vi "Fetch Digital Waveform.vi"(8 "error in (no error)":errorcluster, 9 "Timeout (10000 ms)":u32=10000, 10 "Source (0: POD 1)":u16(ring) items=["POD 1", "POD 2"], 11 "VISA resource name":refnum<visa-resource-name>) -> (0 "error out":errorcluster, 2 "Digital Waveform Graph":digitalwaveform(graph), 3 "VISA resource name out":refnum<visa-resource-name>)   [LabVIEW 2018, in "Agilent 6000 Series.lvlib"]
doc: "Returns the waveform the oscilloscope acquired for the specified channel. The waveform is from an acquisition that you initiate prior to calling this VI.\n\nYou use the Initiate VI to start an acquisition on the channels that you enable with the <B>Configure Digital Channel</B> VI. The oscilloscope acquires waveforms for the enabled channels concurrently. You must call this VI separately for each enabled channel to obtain the waveforms.\n\nYou can call the <B>Read Digital Waveform</B> VI instead of using low level VIs.\n\n<B>NOTE:</B>\n\n1. This VI is only supported by MSO models; running this VI with a DSO model might throw an error.\n\n2. This VI does not check the instrument status. Typically, you call this VI only in a sequence of calls to other low-level instrument driver VIs. The sequence performs one operation. You use the low-level VIs to optimize one or more aspects of interaction with the instrument."
uses:
  Agilent 6000 Series.lvlib
  <vilib>/Waveform/DWDTOps.llb/DWDT Boolean Array to Digital.vi
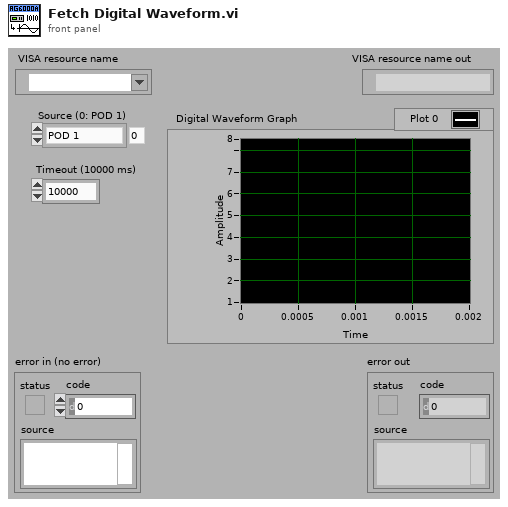
[diagram p1: front panel]
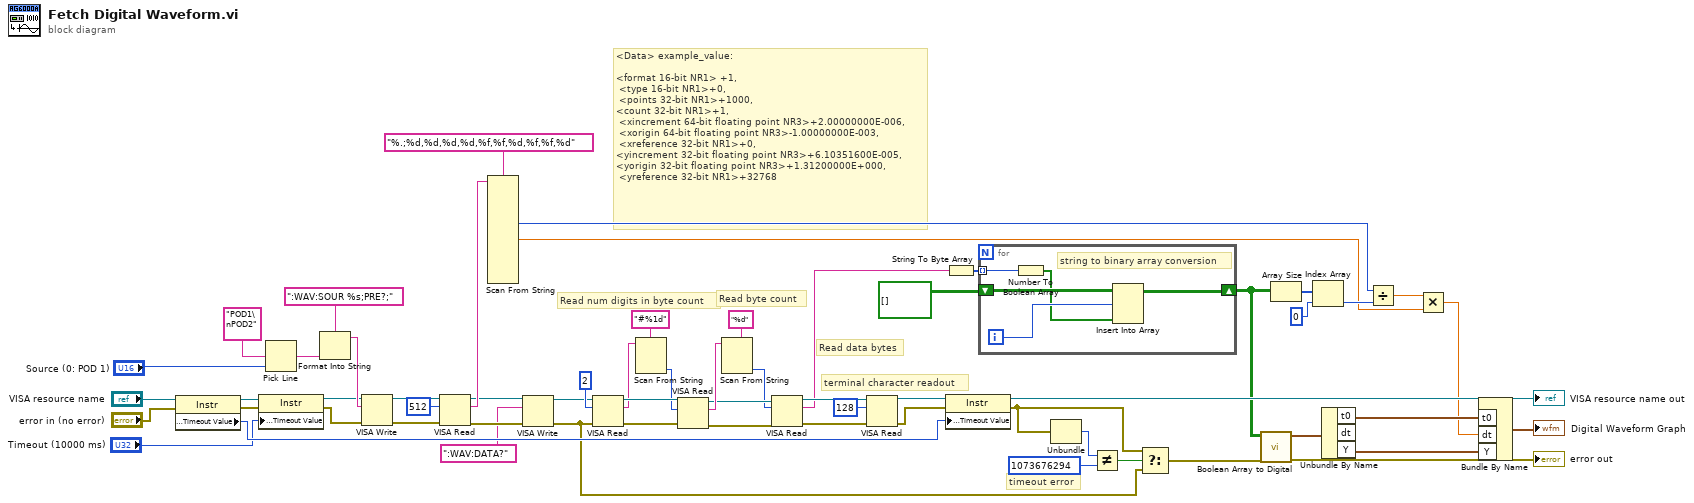
[diagram p0: block diagram]
diagram:
  # "timeout error"
  # "<Data> example_value:\n\n<format 16-bit NR1> +1,\n <type 16-bit NR1>+0,\n <points 32-bit NR1>+1000, \n<count 32-bit NR1>+1,\n <xincrement 64-bit floating point NR3>+2.00000000E-006,\n <xorigin 64-bit floating point NR3>-1.00000000E-003,\n <xreference 32-bit NR1>+0, \n<yincrement 32-bit floating point NR3>+6.10351600E-005, \n<yorigin 32-bit floating point NR3>+1.31200000E+000,\n <yreference 32-bit NR1>+32768"
  # "terminal character readout"
  # "Read data bytes"
  # "Read num digits in byte count"
  # "Read byte count"
  n1 = property on="Property Node" class="Instr"(reference="VISA resource name", error in="error in (no error)") -> (reference out=w49:refnum<visa-resource-name>, error out=w48:errorcluster, "General Settings:Timeout Value"=w50:u32)
  n2 = property on="Property Node" class="Instr"(reference=w49, error in=w48, "General Settings:Timeout Value"="Timeout (10000 ms)") -> (reference out=w46:refnum<visa-resource-name>, error out=w45:errorcluster)
  n3 = Pick Line(multi-line string="POD1\nPOD2", line index="Source (0: POD 1)") -> (output string=w58:string)  [unwired: 1 in]
  n4 = Format Into String(format string=":WAV:SOUR %s;PRE?;", w58) -> (resulting string=w57:string)  [unwired: 2 in, 1 out]
  n5 = VISA Write(VISA resource name=w46, write buffer=w57, error in (no error)=w45) -> (VISA resource name out=w55:refnum<visa-resource-name>, error out=w56:errorcluster)  [unwired: 1 out]
  n6 = VISA Read(VISA resource name=w55, byte count=u32 512, error in (no error)=w56) -> (VISA resource name out=w44:refnum<visa-resource-name>, read buffer=w53:string, error out=w43:errorcluster)  [unwired: 1 out]
  n7 = Scan From String(format string="%.;%d,%d,%d,%d,%f,%f,%d,%f,%f,%d", input string=w53) -> (output 3=w4:i32, output 5=w2:dbl)  [unwired: 20 in, 3 out]
  n8 = VISA Write(VISA resource name=w44, write buffer=":WAV:DATA?", error in (no error)=w43) -> (VISA resource name out=w35:refnum<visa-resource-name>, error out=w19:errorcluster)  [unwired: 1 out]
  n9 = VISA Read(VISA resource name=w35, byte count=u32 2, error in (no error)=w19) -> (VISA resource name out=w38:refnum<visa-resource-name>, read buffer=w36:string, error out=w39:errorcluster)  [unwired: 1 out]
  n10 = Scan From String(format string="#%1d", input string=w36) -> (output 1=w37:i32)  [unwired: 3 in, 3 out]
  n11 = VISA Read(VISA resource name=w38, byte count=w37, error in (no error)=w39) -> (VISA resource name out=w31:refnum<visa-resource-name>, read buffer=w33:string, error out=w32:errorcluster)  [unwired: 1 out]
  n12 = Scan From String(format string="%d", input string=w33) -> (output 1=w30:i32)  [unwired: 3 in, 3 out]
  n13 = VISA Read(VISA resource name=w31, byte count=w30, error in (no error)=w32) -> (VISA resource name out=w28:refnum<visa-resource-name>, read buffer=w16:string, error out=w29:errorcluster)  [unwired: 1 out]
  n14 = VISA Read(VISA resource name=w28, byte count=u32 128, error in (no error)=w29) -> (VISA resource name out=w27:refnum<visa-resource-name>, error out=w26:errorcluster)  [unwired: 2 out]
  n15 = String To Byte Array(string=w16) -> (unsigned byte array=w18:u8[])
  n16 = property on="Property Node" class="Instr"(reference=w27, error in=w26, "General Settings:Timeout Value"=w50) -> (reference out=→"VISA resource name out":refnum<visa-resource-name>, error out=w21:errorcluster)
  n17 = for {
    tunnel: w18 -> [w66] mode=indexing
    shift-right: [w64] -> w8
    shift-left: bool[][] [] ("boolean array") -> [w65]
    i -> [w63]
    # "string to binary array conversion"
    n18 = Number To Boolean Array(number=w66) -> (Boolean array=w62:bool[])
    n19 = Insert Into Array(array=w65, index (row)=w63, new element=w62) -> (w64:bool[][])  [unwired: 1 in]
  }
  n20 = Unbundle(w21) -> ("code"=w24:i32)  [unwired: 2 out]
  n21 = Not Equal?(x=w24, y=1073676294) -> (x != y?=w22:bool)
  n22 = Select(t=w21, s=w22, f=w19) -> (s? t:f=w14:errorcluster)
  n23 = call-poly <vilib>:"Boolean Array to Digital.vi"("error in (no error)"=w14, "boolean array"=w8) -> ("error out"=→"error out":errorcluster, "digital waveform"=w12:digitalwaveform)  [unwired: 8 in]
  n24 = Array Size(array=w8) -> (size(s)=w7:i32[])
  n25 = Index Array(array=w7, index=0) -> (element=w5:i32)
  n26 = Unbundle By Name ("Get Waveform Components")(w12) -> ("t0"=w10:timestamp, "Y"=w11:digitaldata)  [unwired: 1 out]
  n27 = Divide(x=w4, y=w5) -> (x/y=w3:dbl)
  n28 = Multiply(x=w3, y=w2) -> (x*y=w1:dbl)
  n29 = Bundle By Name ("Build Waveform")("t0"=w10, "dt"=w1, "Y"=w11) -> (→"Digital Waveform Graph":digitalwaveform)  [unwired: 1 in]
